vi "SVT Get Spectrum Subset (N Ch).vi"(0 "spectra":cluster{"x0":dbl, "dx":dbl, "magnitude":dbl[]}[](array[cluster]) {"magnitude" format="%.2f"; "dx" format="%.2f"; "x0" format="%.2f"}, 2 "range":cluster{"start":dbl, "stop":dbl}={"start"=-1.0, "stop"=-1.0} {"stop" format="%.2f"; "start" format="%.2f"}, 4 "spectrum info":T1[](array[typedef]) {"x-axis units" items=["Time (s)"=0, "Frequency-CB (Hz)"=1, "Frequency-CPB (Hz)"=1248, "Frequency-Arbitrary (Hz)"=2357, "Quefrency (s)"=2, "Revolutions (rev)"=3, "Order"=4, "Speed (RPM)"=11, "Speed (rad/s)"=21, "Index"=65535]; "weighting filter" items=["Linear", "A-weighting", "B-weighting", "C-weighting", "ITU-R 468-4", "Dolby", "CCITT", "C-message", "Wb", "Wc", "Wd", "We", "Wf", "Wh", "Wj", "Wk", "Wm", "AES17 20 kHz lowpass", "AES17 40 kHz lowpass", "AES17 20 kHz highpass", "AES17 40 kHz highpass"]; "dB reference [EU]" format="%.2f"; "engineering units" items=["custom..."=0, "V"=1, "A"=21, "C"=30, "pC"=31, "s"=32, "-"=29, "Pa"=2, "N"=20, "g"=3, "m/s^2"=4, "m/s"=5, "m"=6, "mm/s"=12, "mm"=13, "micron/s"=14, "micron"=15, "in/s^2"=7, "in/s"=8, "in"=9, "mil/s"=10, "mil"=11, "rad/s^2"=16, "rad/s"=17, "rad"=18, "deg/s^2"=26, "deg/s"=27, "deg"=28, "RPM"=22, "cycle/s^2"=23, "Hz"=24, "cycle"=25, "strain"=19]; "spectral info"."window" items=["None "=0, "Hanning"=1, "Hamming"=2, "Blackman-Harris"=3, "Exact Blackman"=4, "Blackman"=5, "Flat Top"=6, "4 Term B-Harris "=7, "7 Term B-Harris"=8, "Low Sidelobe"=9, "Force - Exponential"=10, "Gaussian"=62]}, 5 "error in (no error)":errorcluster) -> (14 "spectra subsets":cluster{"x0":dbl, "dx":dbl, "magnitude":dbl[]}[](array[cluster]) {"magnitude" format="%.2f"; "dx" format="%.2f"; "x0" format="%.2f"}, 15 "unit labels":string[](array[string]), 16 "actual ranges":cluster{"start":dbl, "stop":dbl}[](array[cluster]) {"stop" format="%.2f"; "start" format="%.2f"}, 17 "range labels":string[](array[string]), 18 "dup spectrum info":T1[](array[typedef]) {"x-axis units" items=["Time (s)"=0, "Frequency-CB (Hz)"=1, "Frequency-CPB (Hz)"=1248, "Frequency-Arbitrary (Hz)"=2357, "Quefrency (s)"=2, "Revolutions (rev)"=3, "Order"=4, "Speed (RPM)"=11, "Speed (rad/s)"=21, "Index"=65535]; "weighting filter" items=["Linear", "A-weighting", "B-weighting", "C-weighting", "ITU-R 468-4", "Dolby", "CCITT", "C-message", "Wb", "Wc", "Wd", "We", "Wf", "Wh", "Wj", "Wk", "Wm", "AES17 20 kHz lowpass", "AES17 40 kHz lowpass", "AES17 20 kHz highpass", "AES17 40 kHz highpass"]; "dB reference [EU]" format="%.2f"; "engineering units" items=["custom..."=0, "V"=1, "A"=21, "C"=30, "pC"=31, "s"=32, "-"=29, "Pa"=2, "N"=20, "g"=3, "m/s^2"=4, "m/s"=5, "m"=6, "mm/s"=12, "mm"=13, "micron/s"=14, "micron"=15, "in/s^2"=7, "in/s"=8, "in"=9, "mil/s"=10, "mil"=11, "rad/s^2"=16, "rad/s"=17, "rad"=18, "deg/s^2"=26, "deg/s"=27, "deg"=28, "RPM"=22, "cycle/s^2"=23, "Hz"=24, "cycle"=25, "strain"=19]; "spectral info"."window" items=["None "=0, "Hanning"=1, "Hamming"=2, "Blackman-Harris"=3, "Exact Blackman"=4, "Blackman"=5, "Flat Top"=6, "4 Term B-Harris "=7, "7 Term B-Harris"=8, "Low Sidelobe"=9, "Force - Exponential"=10, "Gaussian"=62]}, 19 "error out":errorcluster)   [LabVIEW 2017]
doc: "Extracts the subset of the spectrum specified by <B>range</B>. <B>x0</B> is updated to reflect the new start frequency, <B>dx</B> is the same as in the input spectrum, and the spectrum array is shortened so the last element corresponds with the stop value specified in the <B>range</B>. Use this VI for operations such as limiting subsequent spectrum operations to the region of interest or removing the part of the spectrum outside the alias-free bandwidth, as well as others. You can use this polymorphic VI to take a subset of a single spectrum, N spectra, a single complex spectrum, or N complex spectra. The data type you wire to the <B>phase spectrum</B> input determines the polymorphic instance to use."
uses:
  <vilib>/addons/_NISVFA/_Shared subVIs/Controls/svc_Spectrum Info.ctl
  <vilib>/addons/_NISVFA/_Shared subVIs/Controls/svc_X-Axis Units.ctl
  <vilib>/addons/_NISVFA/_Shared subVIs/Controls/svc_Spectrum Type.ctl
  <vilib>/addons/_NISVFA/_Shared subVIs/Controls/svc_Engineering Units Text Ring.ctl
  <vilib>/addons/_NISVFA/_Shared subVIs/Controls/svc_Weighting Filter Text Ring.ctl
  <vilib>/addons/_NISVFA/_Shared subVIs/Controls/svc_Complimentary Spectrum Units.ctl
  <vilib>/addons/_NISVFA/_Shared subVIs/Common/svc_Spectrum Units.vi
  <vilib>/addons/_NISVFA/_Shared subVIs/Common/svc_Build Unit Label for Frequency Range.vi
  <vilib>/addons/_NISVFA/_Shared subVIs/Common/svc_Convert Frequency to Frequency String.vi
  <vilib>/addons/_NISVFA/_Shared subVIs/Common/svc_Check Frequency Range in Spectrum.vi
  <vilib>/addons/_NISVFA/_Shared subVIs/Common/svc_Get Weighting Enum and Labels.vi
  <vilib>/addons/_NISVFA/_Shared subVIs/Common/svc_Unit Label Lexical Class.vi
  <vilib>/addons/_NISVFA/_Shared subVIs/Common/svc_Engineering Units to Unit Label.vi
  <vilib>/addons/_NISVFA/_Shared subVIs/Common/svc_Format Value (DBL).vi
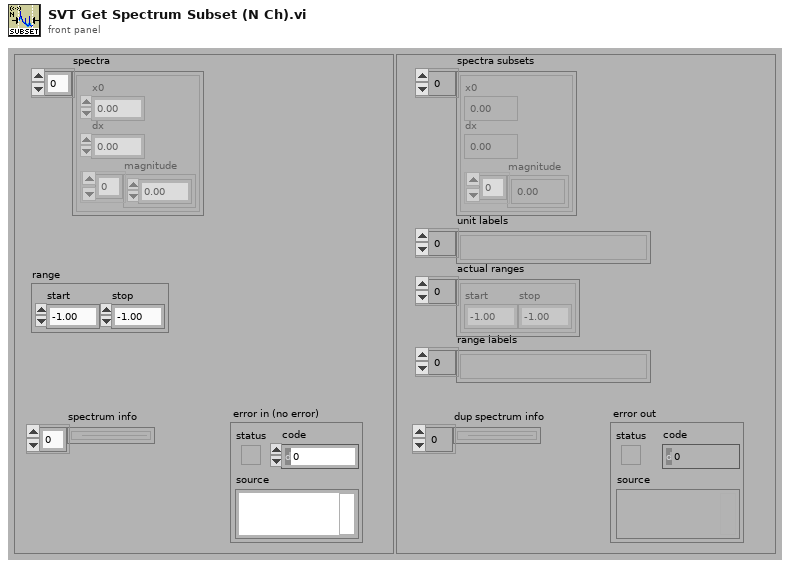
[diagram p1: front panel]
types:
  T1 = typedef "svc_Spectrum Info.ctl" = cluster{"channel name":string, "description":string, "x-axis units":T2, "spectral info":cluster{"spectrum type":T3, "linear/dB":enum16{"linear", "dB"}, "window":u16, "window size":i32, "FFT size":i32}, "engineering units":T4, "custom label":string, "dB reference [EU]":dbl, "peak units":enum16{"rms", "peak", "peak-peak"}, "weighting filter":T5, "spectral density?":bool, "unit label":string, "spectrum skewed?":bool, "complimentary spectrum units":T6}
  T2 = typedef "svc_X-Axis Units.ctl" = u16
  T3 = typedef "svc_Spectrum Type.ctl" = enum16{"FFT Spectrum [complex]", "Amplitude [Magnitude]", "Power [Magnitude^2]", "Cross Spectrum [complex]", "Frequency Response [Complex]"}
  T4 = typedef "svc_Engineering Units Text Ring.ctl" = u16
  T5 = typedef "svc_Weighting Filter Text Ring.ctl" = u16
  T6 = typedef "svc_Complimentary Spectrum Units.ctl" = enum16{"none", "radians", "degrees", "cycles", "imaginary"}
  T7 = cluster{"start frequency":dbl, "stop frequency":dbl}[]
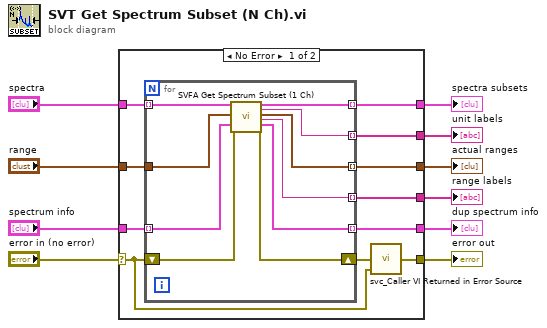
[diagram p0: block diagram]
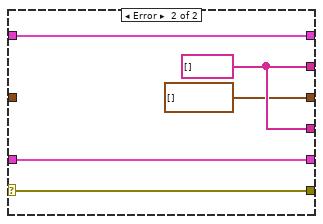
[diagram p2: hidden frame]
diagram:
  n1 = case shown="No Error" "error in (no error)" {
    selector: "error in (no error)" -> [w11 w36]
    tunnel: [w20 w36] -> w10
    tunnel: "spectrum info" -> [w18 w34]
    tunnel: "spectra" -> [w19 w35]
    tunnel: "range" -> [w17 _]
    tunnel: [w16 w35] -> w5
    tunnel: [w15 w34] -> w4
    tunnel: [w14 w33] -> w1
    tunnel: [w13 T7 []] -> w3
    tunnel: [w12 w33] -> w2
    frame No Error {
      n2 = for {
        shift-right: [w25] -> w21
        shift-left: w11 -> [w26]
        tunnel: w19 -> [w31] mode=indexing
        tunnel: w18 -> [w30] mode=indexing
        tunnel: w17 -> [w22]
        tunnel: [w29] -> w16 mode=indexing
        tunnel: [w28] -> w15 mode=indexing
        tunnel: [w27] -> w14 mode=indexing
        tunnel: [w24] -> w13 mode=indexing
        tunnel: [w23] -> w12 mode=indexing
        n3 = call <vilib>:"SVFA Get Spectrum Subset (1 Ch).vi"("spectrum"=w31, "range"=w22, "spectrum info"=w30, "error in (no error)"=w26) -> ("spectrum subset"=w29:cluster{"x0":dbl, "dx":dbl, "magnitude":dbl[]}, "unit label"=w27:string, "actual range"=w24:cluster{"start":dbl, "stop":dbl}, "range label"=w23:string, "dup spectrum info"=w28:T1, "error out"=w25:errorcluster)  [unwired: 10 in]
      }
      n4 = call <vilib>:"svc_Caller VI Returned in Error Source.vi"("warning input to caller"=w11, "error in (no error)"=w21) -> ("error out"=w20:errorcluster)  [unwired: 3 in]
    }
    frame Error {
      w33 = string[] []
    }
  }
  "error out" <- w10
  "spectra subsets" <- w5
  "dup spectrum info" <- w4
  "range labels" <- w2
  "unit labels" <- w1
  "actual ranges" <- w3
